vi "MALT Global.vi"() -> ()   [LabVIEW 2018, in "AltonTech MALT200817.lvlib"]
uses:
  AltonTech MALT200817.lvlib
panel:
  in  "Parameters":T1
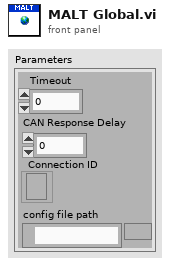
[diagram p1: front panel]
types:
  T1 = cluster{"Timeout":i32, "CAN Response Delay":i32, "Connection ID":refnum<k5>, "config file path":path}
diagram:
